vi "Run_Pre Core.vi"(0 "While Loop in":refnum<class "While Loop.lvclass">, 11 "error in (no error)":errorcluster) -> (4 "While Loop out":refnum<class "While Loop.lvclass">, 6 "Execute Run Core?":bool, 15 "error out":errorcluster)   [LabVIEW 2016, in "While Loop.lvclass"]
uses:
  While Loop.lvclass
  While Loop.lvclass/While Loop.ctl
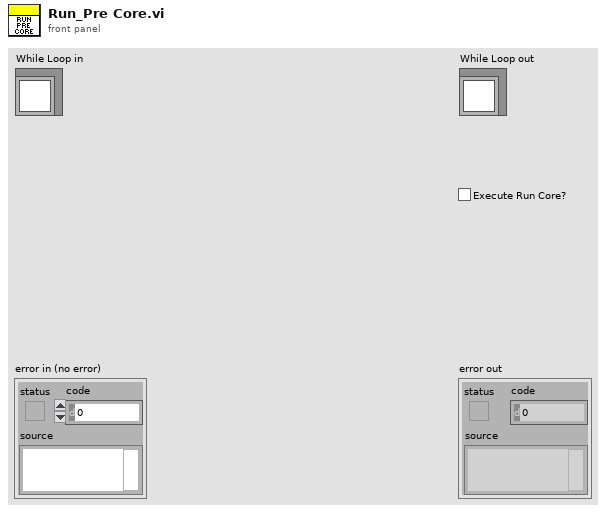
[diagram p1: front panel]
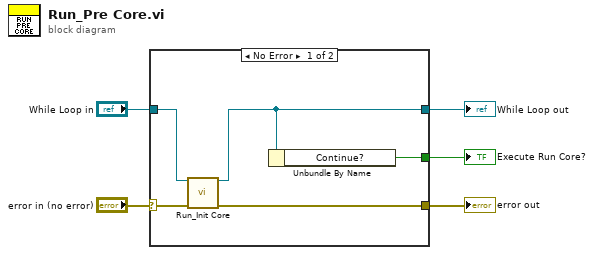
[diagram p0: block diagram]
diagram:
  n1 = case shown="No Error" "error in (no error)" {
    selector: "error in (no error)" -> [w9 w12]
    tunnel: "While Loop in" -> [w7 w11]
    tunnel: [w10 _] -> w4
    tunnel: [w6 w11] -> w3
    tunnel: [w8 w12] -> w1
    frame No Error {
      n2 = call-dynamic "Run_Init Core.vi"("functionbase in"=w7, "error in (no error)"=w9) -> ("functionbase out"=w6:refnum<class "While Loop.lvclass">, "error out"=w8:errorcluster)  [unwired: 12 in]
      n3 = Unbundle By Name(w6) -> ("Continue?"=w10:bool)
    }
    frame Error {
    }
  }
  "error out" <- w1
  "While Loop out" <- w3
  "Execute Run Core?" <- w4
